vi "Convert TDM to TDMS.vi"(6 "data chunk size":u32=10000000 format="%.0e", 7 "view new file?":bool, 8 "error in (no error)":errorcluster, 9 "target file operation (2:create or replace)":T1(ring)=enum."create or replace", 10 "target file path (*.tdms)":path, 11 "source file path (*.tdm)":path) -> (0 "error out":errorcluster, 2 "target file path (*.tdms) out":path, 3 "source file path (*.tdm) out":path)   [LabVIEW 2020]
doc: "LabVIEW no longer supports this VI. Use the Convert to TDM or TDMS VI instead.\n\nConverts the specified file from the .tdm file format to the .tdms file format."
uses:
  <vilib>/Platform/storage/lvStorage.llb/_openFunction.ctl
  <vilib>/Platform/storage/Storage.llb/Get Property (Storage Refnums).vi
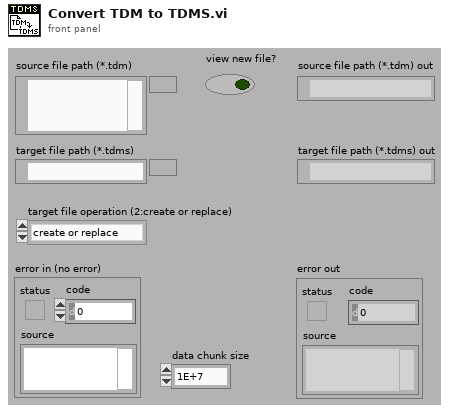
[diagram p1: front panel]
types:
  T1 = enum16{"open", "open or create", "create or replace", "create", "open (read-only)"}
  T2 = typedef "_openFunction.ctl" = enum16{"open", "open or create", "create or replace", "create", "open (read only)"}
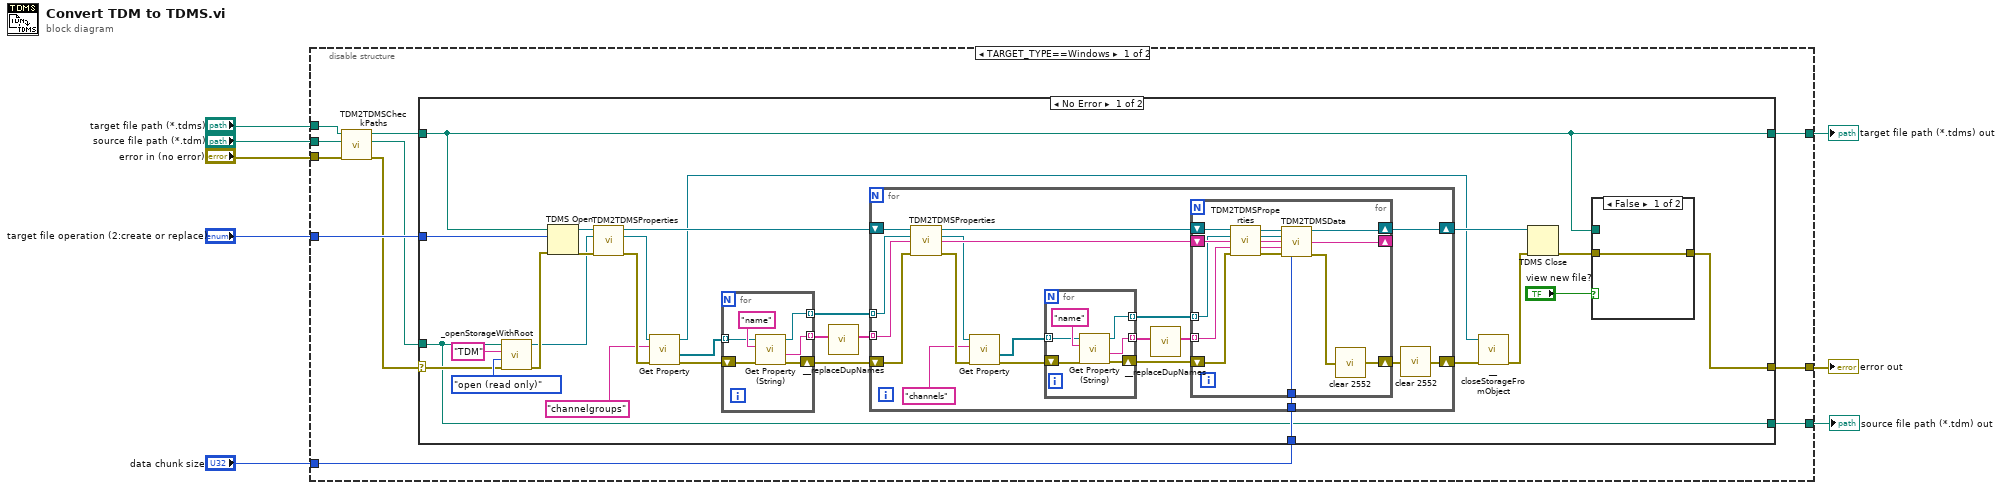
[diagram p0: block diagram]
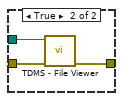
[diagram p2: hidden frame]
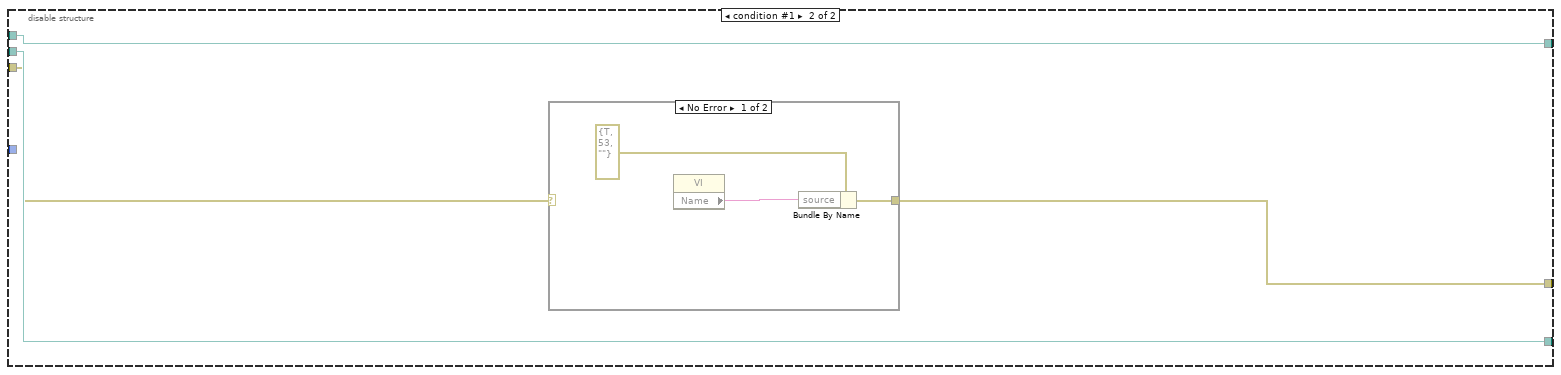
[diagram p4: hidden frame]
diagram:
  n1 = disable-structure shown="TARGET_TYPE==Windows" {
    disable-tunnel: "target file operation (2:create or replace)" -> [w19 _]
    disable-tunnel: [w18 w101] -> w7
    disable-tunnel: [w16 w104] -> w6
    disable-tunnel: "source file path (*.tdm)" -> [w15 w103]
    disable-tunnel: [w13 w103] -> w4
    disable-tunnel: "data chunk size" -> [w12 _]
    disable-tunnel: "error in (no error)" -> [w11 w102]
    disable-tunnel: "target file path (*.tdms)" -> [w10 w104]
    frame condition #0 (active) {
      n2 = call <vilib>:"TDM2TDMSCheckPaths.vi"("error in (no error)"=w11, "TDM Path In"=w15, "New TDMS Path In"=w10) -> ("error out"=w14:errorcluster, "TDM File Out"=w9:path, "TDMS File Out"=w17:path)  [unwired: 6 in]
      n3 = case shown="No Error" w14 {
        selector: w14 -> [w36 w98]
        tunnel: w19 -> [w45 _]
        tunnel: [w20 w98] -> w18
        tunnel: w9 -> [w33 w99]
        tunnel: w17 -> [w32 w100]
        tunnel: [w32 w100] -> w16
        tunnel: [w33 w99] -> w13
        tunnel: w12 -> [w34 _]
        frame No Error {
          n4 = call <vilib>:"_openStorageWithRoot.vi"("error in (no error)"=w36, "Overwrite Options"=_openFunction."open (read only)", "Storage Format"="TDM", "Storage Location"=w33) -> ("error out"=w35:errorcluster, "Data Object"=w27:refnum<k20>)  [unwired: 6 in]
          n5 = TDMS Open(8:w35, 10:w45, 11:w32) -> (0:w47:errorcluster, 3:w44:refnum<k34>)  [unwired: 4 in]
          n6 = call <vilib>:"TDM2TDMSProperties.vi"("tdms file in"=w44, "Data Object in"=w27, "error in (no error)"=w47) -> ("tdms file out"=w46:refnum<k34>, "Data Object out"=w31:refnum<k20>, "error out"=w30:errorcluster)  [unwired: 8 in, 2 out]
          n7 = call-poly <vilib>:"Get Property.vi"("error in (no error)"=w30, "Property name"="channelgroups", "storage refnum"=w31) -> ("error out"=w26:errorcluster, "Value"=w25:refnum<k20>[], "storage refnum out"=w29:refnum<k20>)  [unwired: 6 in]
          n8 = for {
            shift-right: [w52] -> w23
            shift-left: w26 -> [w51]
            tunnel: w25 -> [w50] mode=indexing
            tunnel: [w49] -> w24 mode=indexing
            tunnel: [w48] -> w22 mode=indexing
            n9 = call <vilib>:"Get Property (String).vi"("error in (no error)"=w51, "Property name"="name", "storage refnum"=w50) -> ("error out"=w52:errorcluster, "Value"=w48:string, "storage refnum out"=w49:refnum<k20>)  [unwired: 6 in]
          }
          n10 = call <vilib>:"__replaceDupNames.vi"("input names"=w22) -> ("output names"=w21:string[])  [unwired: 10 in]
          n11 = for {
            shift-right: [w74] -> w37
            shift-left: w46 -> [w76]
            shift-right: [w59] -> w41
            shift-left: w23 -> [w61]
            tunnel: w34 -> [w72]
            tunnel: w24 -> [w60] mode=indexing
            tunnel: w21 -> [w62] mode=indexing
            n12 = call <vilib>:"TDM2TDMSProperties.vi"("tdms file in"=w76, "Data Object in"=w60, "group name"=w62, "error in (no error)"=w61) -> ("tdms file out"=w75:refnum<k34>, "Data Object out"=w69:refnum<k20>, "group name out"=w73:string, "error out"=w71:errorcluster)  [unwired: 7 in, 1 out]
            n13 = call-poly <vilib>:"Get Property.vi"("error in (no error)"=w71, "Property name"="channels", "storage refnum"=w69) -> ("error out"=w68:errorcluster, "Value"=w67:refnum<k20>[])  [unwired: 6 in, 1 out]
            n14 = for {
              shift-right: [w80] -> w66
              shift-left: w68 -> [w81]
              tunnel: w67 -> [w79] mode=indexing
              tunnel: [w78] -> w65 mode=indexing
              tunnel: [w77] -> w63 mode=indexing
              n15 = call <vilib>:"Get Property (String).vi"("error in (no error)"=w81, "Property name"="name", "storage refnum"=w79) -> ("error out"=w80:errorcluster, "Value"=w78:string, "storage refnum out"=w77:refnum<k20>)  [unwired: 6 in]
            }
            n16 = call <vilib>:"__replaceDupNames.vi"("input names"=w65) -> ("output names"=w64:string[])  [unwired: 10 in]
            n17 = for {
              shift-right: [w93] -> w74
              shift-left: w75 -> [w96]
              shift-right: [w83] -> w58
              shift-left: w66 -> [w86]
              tunnel: w72 -> [w89]
              shift-right: [w88] -> _
              shift-left: w73 -> [w97]
              tunnel: w64 -> [w85] mode=indexing
              tunnel: w63 -> [w87] mode=indexing
              n18 = call <vilib>:"TDM2TDMSProperties.vi"("tdms file in"=w96, "Data Object in"=w87, "group name"=w97, "channel name"=w85, "error in (no error)"=w86) -> ("tdms file out"=w95:refnum<k34>, "Data Object out"=w94:refnum<k20>, "group name out"=w91:string, "channel name out"=w90:string, "error out"=w92:errorcluster)  [unwired: 6 in]
              n19 = call <vilib>:"TDM2TDMSData.vi"("tdms file in"=w95, "storage refnum in"=w94, "group name"=w91, "channel name"=w90, "error in (no error)"=w92, "chunk size"=w89) -> ("tdms file out"=w93:refnum<k34>, "group name out"=w88:string, "error out"=w84:errorcluster)  [unwired: 5 in, 2 out]
              n20 = call <vilib>:"clear 2552.vi"("error in"=w84) -> ("error out"=w83:errorcluster)
            }
            n21 = call <vilib>:"clear 2552.vi"("error in"=w58) -> ("error out"=w59:errorcluster)
          }
          n22 = call <vilib>:"__closeStorageFromObject.vi"("error in (no error)"=w41, "storage refnum"=w29) -> ("error out"=w40:errorcluster)  [unwired: 5 in]
          n23 = TDMS Close(8:w40, 11:w37) -> (0:w43:errorcluster)  [unwired: 1 out]
          n24 = case shown="False" "view new file?" {
            tunnel: w43 -> [w54 w57]
            tunnel: [w54 w56] -> w20
            tunnel: w32 -> [_ w55]
            frame False {
            }
            frame True {
              n25 = call <vilib>:"TDMS - File Viewer.vi"("error in (no error)"=w57, "file path"=w55) -> ("error out"=w56:errorcluster)  [unwired: 4 in, 1 out]
            }
          }
        }
        frame Error {
        }
      }
    }
    frame condition #1 {
      n26 = case shown="No Error" w102 {
        selector: w102 -> [_ w108]
        tunnel: [w106 w108] -> w101
        frame No Error {
          n27 = property class="VI"() -> ("Name"=w105:string)  [unwired: 2 in, 2 out]
          n28 = Bundle By Name(cluster=errorcluster {"status"=TRUE, "code"=53, "source"=""} ("error IO"), "source"=w105) -> (w106:errorcluster)
        }
        frame Error {
        }
      }
    }
  }
  "error out" <- w7
  "target file path (*.tdms) out" <- w6
  "source file path (*.tdm) out" <- w4
